vi "List Band.vi"(6 "Low Limit (0.0)":dbl min=0.0 max=9.9e+37 step=1.0 format="%.4f", 7 "High Limit (0.0)":dbl min=0.0 max=9.9e+37 step=1.0 format="%.4f", 8 "error in (no error)":errorcluster, 9 "Imp Parameter (0: A)":u32(slide) max=2 step=1, 10 "Sweep Point Num (1)":i16=1 min=1 max=10 step=1, 11 "VISA resource name":refnum<visa-resource-name>) -> (0 "error out":errorcluster, 3 "VISA resource name out":refnum<visa-resource-name>)   [LabVIEW 2015, in "Agilent 428X Series.lvlib"]
doc: "This function sets the limit values of the limit function for the list sweep measurement."
uses:
  <instrlib>/Agilent 428X Series/Agilent 428X Series.lvlib
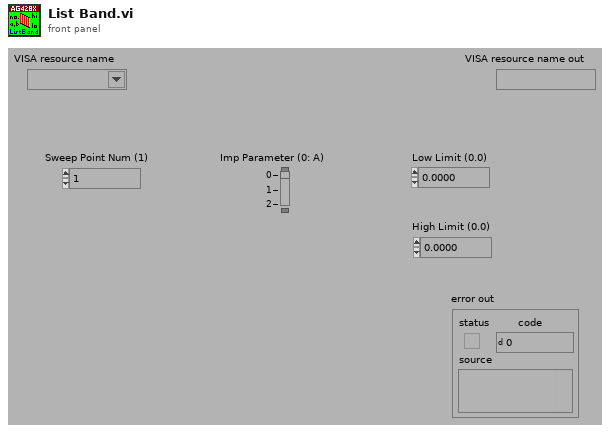
[diagram p1: front panel]
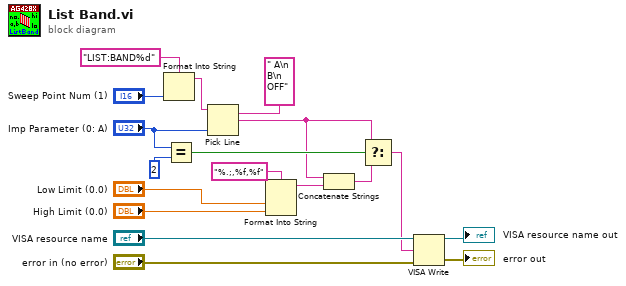
[diagram p0: block diagram]
diagram:
  n1 = Format Into String(format string="LIST:BAND%d", "Sweep Point Num (1)") -> (resulting string=w13:string)  [unwired: 2 in, 1 out]
  n2 = Equal?(x="Imp Parameter (0: A)", y=u32 2) -> (x = y?=w6:bool)
  n3 = Pick Line(string ("")=w13, multi-line string=" A\n B\n OFF", line index="Imp Parameter (0: A)") -> (output string=w4:string)
  n4 = Format Into String(format string="%.;,%f,%f", "Low Limit (0.0)", "High Limit (0.0)") -> (resulting string=w3:string)  [unwired: 2 in, 1 out]
  n5 = Concatenate Strings(w4, w3) -> (w2:string)
  n6 = Select(t=w4, s=w6, f=w2) -> (s? t:f=w1:string)
  n7 = VISA Write(VISA resource name="VISA resource name", write buffer=w1, error in (no error)="error in (no error)") -> (VISA resource name out=→"VISA resource name out":refnum<visa-resource-name>, error out=→"error out":errorcluster)  [unwired: 1 out]
